vi "CLSUIP_ClearBlockDiagram_BuildDontDeleteList.vi"(8 "Error In":errorcluster, 11 "VI Refnum In":refnum<vi>) -> (0 "Error Out":errorcluster, 2 "Ctls which must not be deleted.":refnum<vi>[](array[refnum]), 3 "VI Refnum Out":refnum<vi>)   [LabVIEW 2021]
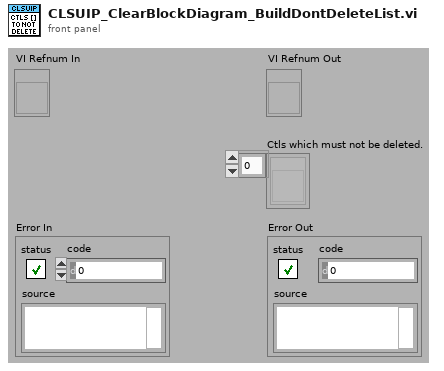
[diagram p1: front panel]
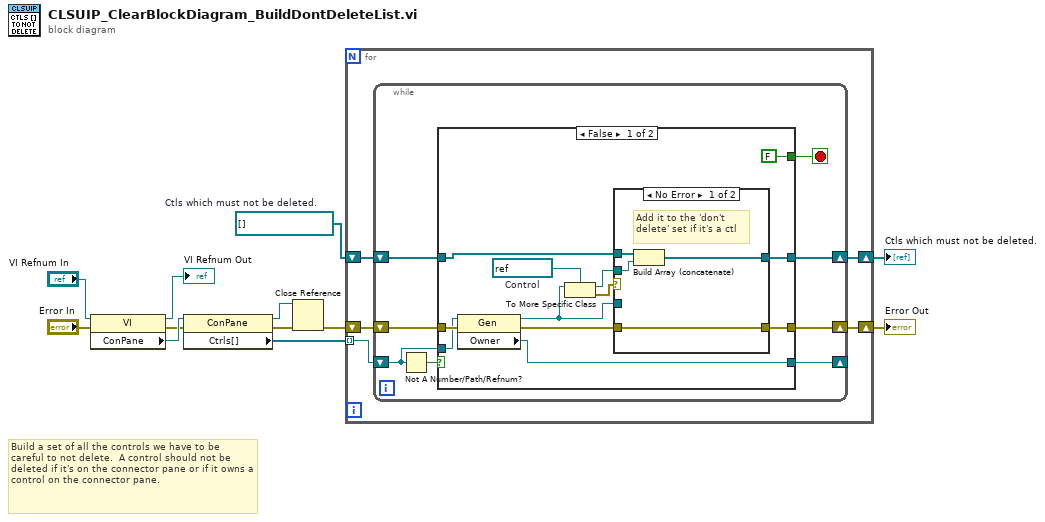
[diagram p0: block diagram]
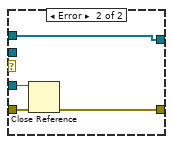
[diagram p2: hidden frame]
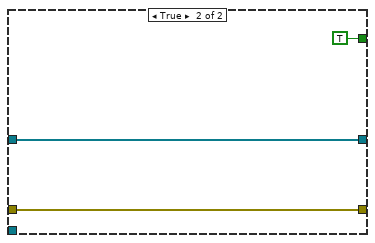
[diagram p3: hidden frame]
diagram:
  w11 = refnum<vi>[] []  # Ctls which must not be deleted.
  # "Build a set of all the controls we have to be careful to not delete.  A control should not be deleted if it's on the connector pane or if it owns a control on the connector pane."
  n1 = property on="Property Node" class="VI"(reference="VI Refnum In", error in="Error In") -> (reference out=→"VI Refnum Out":refnum<vi>, error out=w7:errorcluster, "ConPane"=w9:refnum<vi>)
  n2 = property on="Property Node" class="ConPane"(reference=w9, error in=w7) -> (reference out=w6:refnum<vi>, error out=w5:errorcluster, "Ctrls[]"=w2:refnum<vi>[])
  n3 = Close Reference(reference=w6, error in (no error)=w5) -> (error out=w3:errorcluster)
  n4 = for {
    shift-right: [w17] -> w1
    shift-left: w3 -> [w16]
    tunnel: w2 -> [w13] mode=indexing
    shift-right: [w15] -> w12
    shift-left: w11 -> [w14]
    n5 = while {
      shift-right: [w23] -> w17
      shift-left: w16 -> [w22]
      shift-right: [w21] -> w15
      shift-left: w14 -> [w24]
      shift-right: [w19] -> _
      shift-left: w13 -> [w18]
      stop <- w20 stop-if-true
      n6 = Not A Number/Path/Refnum?(number/path/refnum=w18) -> (NaN/Path/Refnum?=w25:bool)
      n7 = case shown="False" w25 {
        tunnel: w24 -> [w37 w47]
        tunnel: [w36 w47] -> w21
        tunnel: [w33 w48] -> w23
        tunnel: w22 -> [w35 w48]
        tunnel: [FALSE TRUE] -> w20
        tunnel: [w32 _] -> w19
        tunnel: w18 -> [w30 _]
        frame False {
          w26 = refnum<vi> refnum  # Control
          n8 = property class="Gen"(reference=w30, error in=w35) -> (reference out=w27:refnum<vi>, error out=w34:errorcluster, "Owner"=w32:refnum<vi>)
          n9 = To More Specific Class(target class=w26, reference=w27) -> (specific class reference=w28:refnum<vi>, error out=w29:errorcluster)  [unwired: 1 in]
          n10 = case shown="No Error" w29 {
            tunnel: [w41 w42] -> w36
            tunnel: w27 -> [_ w44]
            tunnel: [w39 w45] -> w33
            tunnel: w37 -> [w40 w42]
            tunnel: w34 -> [w39 w43]
            tunnel: w28 -> [w38 _]
            frame No Error {
              # "Add it to the 'don't delete' set if it's a ctl"
              n11 = Build Array (concatenate)(w40, w38) -> (w41:refnum<vi>[])
            }
            frame Error {
              n12 = Close Reference(reference=w44, error in (no error)=w43) -> (error out=w45:errorcluster)
            }
          }
        }
        frame True {
        }
      }
    }
  }
  "Error Out" <- w1
  "Ctls which must not be deleted." <- w12
